vi "cno_form constraint vector.vi"(7 "cno data":T1, 9 "OB":dbl[](array[numeric]), 10 "PB":dbl[][](array[numeric]), 11 "P in":dbl[](array[numeric])) -> (1 "norm":dbl, 3 "P out":dbl[](array[numeric]))   [LabVIEW 2014, in "NI_Gmath.lvlib"]
uses:
  NI_Gmath.lvlib
  cno_data.ctl
  Real Matrix Norm.vi
  NI_AALPro.lvlib
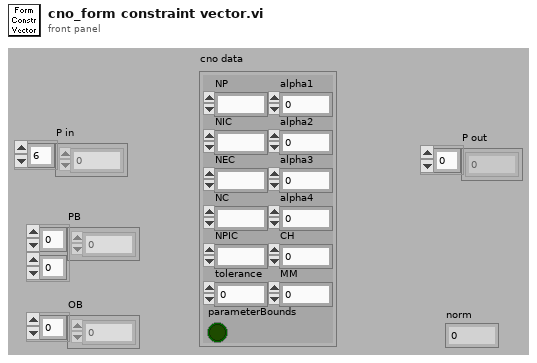
[diagram p1: front panel]
types:
  T1 = typedef "NI_Gmath.lvlib/cno_data.ctl" = cluster{"NP":i32, "NIC":i32, "NEC":i32, "NC":i32, "NPIC":i32, "parameterBounds":bool, "alpha1":dbl, "alpha2":dbl, "alpha3":dbl, "alpha4":dbl, "CH":i32, "MM":i32, "tolerance":dbl}
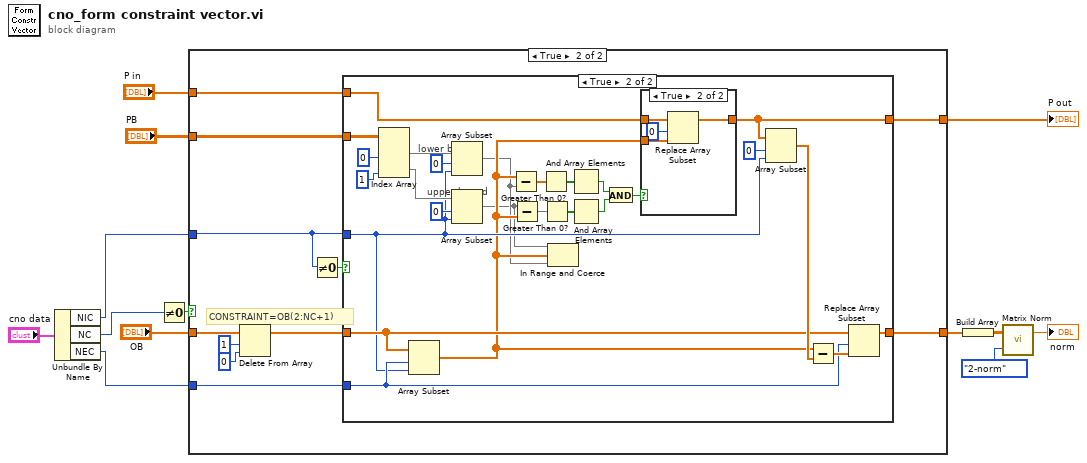
[diagram p0: block diagram]
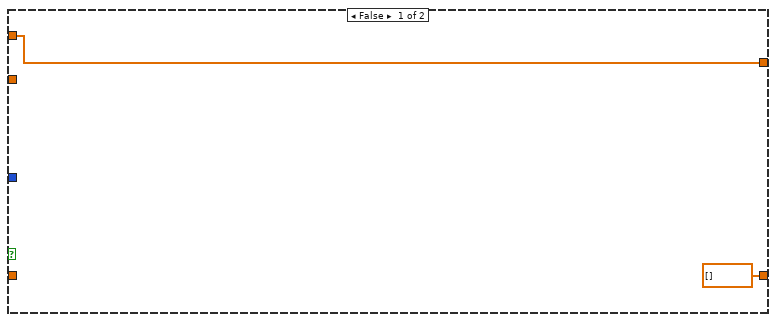
[diagram p2: hidden frame]
diagram:
  n1 = Unbundle By Name("cno data") -> ("NIC"=w3:i32, "NC"=w2:i32, "NEC"=w1:i32)
  n2 = Not Equal To 0?(x=w2) -> (x != 0?=w13:bool)
  n3 = case shown="True" w13 {
    tunnel: "OB" -> [_ w26]
    tunnel: w3 -> [_ w21]
    tunnel: "PB" -> [_ w20]
    tunnel: w1 -> [_ w19]
    tunnel: "P in" -> [w15 w18]
    tunnel: [w15 w17] -> w9
    tunnel: [dbl[] [] ("OB") w16] -> w7
    frame False {
    }
    frame True {
      # "CONSTRAINT=OB(2:NC+1)"
      n4 = Delete From Array(array=w26, length=1, index=0) -> (array with subset deleted=w22:dbl[])  [unwired: 1 out]
      n5 = Not Equal To 0?(x=w21) -> (x != 0?=w23:bool)
      n6 = case shown="True" w23 {
        tunnel: w20 -> [_ w54]
        tunnel: w22 -> [w27 w36]
        tunnel: w21 -> [_ w34]
        tunnel: w19 -> [_ w37]
        tunnel: w18 -> [w28 w41]
        tunnel: [w28 w40] -> w17
        tunnel: [w27 w35] -> w16
        frame False {
        }
        frame True {
          # "upper bound"
          # "lower bound"
          n7 = Index Array(array=w54, index (col) #1=0 ("disabled index (col)"), index (col) #2=1 ("index (col)")) -> (element #1=w51:dbl[], element #2=w50:dbl[])  [unwired: 2 in]
          n8 = Array Subset(array=w36, index=w37, length=w34) -> (w32:dbl[])
          n9 = Array Subset(array=w51, index=0, length=w34) -> (w31:dbl[])
          n10 = Array Subset(array=w50, index=0, length=w34) -> (w30:dbl[])
          n11 = Subtract(x=w32, y=w31) -> (x-y=w47:dbl[])
          n12 = Subtract(x=w30, y=w32) -> (x-y=w46:dbl[])
          n13 = Greater Than 0?(x=w47) -> (x > 0?=w45:bool[])
          n14 = Greater Than 0?(x=w46) -> (x > 0?=w44:bool[])
          n15 = In Range and Coerce(upper limit=w30, x=w32, lower limit=w31) -> ()  [unwired: 2 out]
          n16 = And Array Elements(Boolean array=w45) -> (logical AND=w43:bool)
          n17 = And Array Elements(Boolean array=w44) -> (logical AND=w42:bool)
          n18 = And(x=w43, y=w42) -> (x .and. y?=w29:bool)
          n19 = case shown="True" w29 {
            tunnel: w41 -> [w55 w59]
            tunnel: w32 -> [_ w58]
            tunnel: [w55 w57] -> w40
            frame False {
            }
            frame True {
              n20 = Replace Array Subset(array=w59, new element=w58, index=0) -> (w57:dbl[])
            }
          }
          n21 = Array Subset(array=w40, index=0, length=w34) -> (w39:dbl[])
          n22 = Subtract(x=w32, y=w39) -> (x-y=w38:dbl[])
          n23 = Replace Array Subset(array=w36, new element=w38, index=w37) -> (w35:dbl[])
        }
      }
    }
  }
  "P out" <- w9
  n24 = Build Array(w7) -> (w6:dbl[][])
  n25 = call-poly "Matrix Norm.vi"("norm type"=enum32{"2-norm", "1-norm", "F-norm", "inf-norm"}."2-norm", "Input Matrix"=w6) -> ("norm"=→"norm":dbl)  [unwired: 1 out]
